vi "Mathcad 15 write file.vi"(8 "error in":errorcluster, 11 "DesignRequest":T1={"Project Folder"=path "", "Method Name"="", "Inputs"=[{"Label.Text"="L.Box", "Control Type"=0, "Numeric"=5.0, "Array"=[], "status"=FALSE, "Str Array"=[], "String"="", "unit"="m"}, {"Label.Text"="W.Box", "Control Type"=0, "Numeric"=2.0, "Array"=[], "status"=FALSE, "Str Array"=[], "String"="", "unit"="m"}, {"Label.Text"="H.Box", "Control Type"=0, "Numeric"=11.0, "Array"=[], "status"=FALSE, "Str Array"=[], "String"="", "unit"="m"}], "Version"=0}) -> (0 "error out":errorcluster, 3 "Mathcad w inputs":path)   [LabVIEW 2012, in "Design Server.lvlib"]
uses:
  Design Server.lvlib
  Design Request.ctl
  Variable cluster.ctl
  Folders.ctl
panel:
  out "file text":string
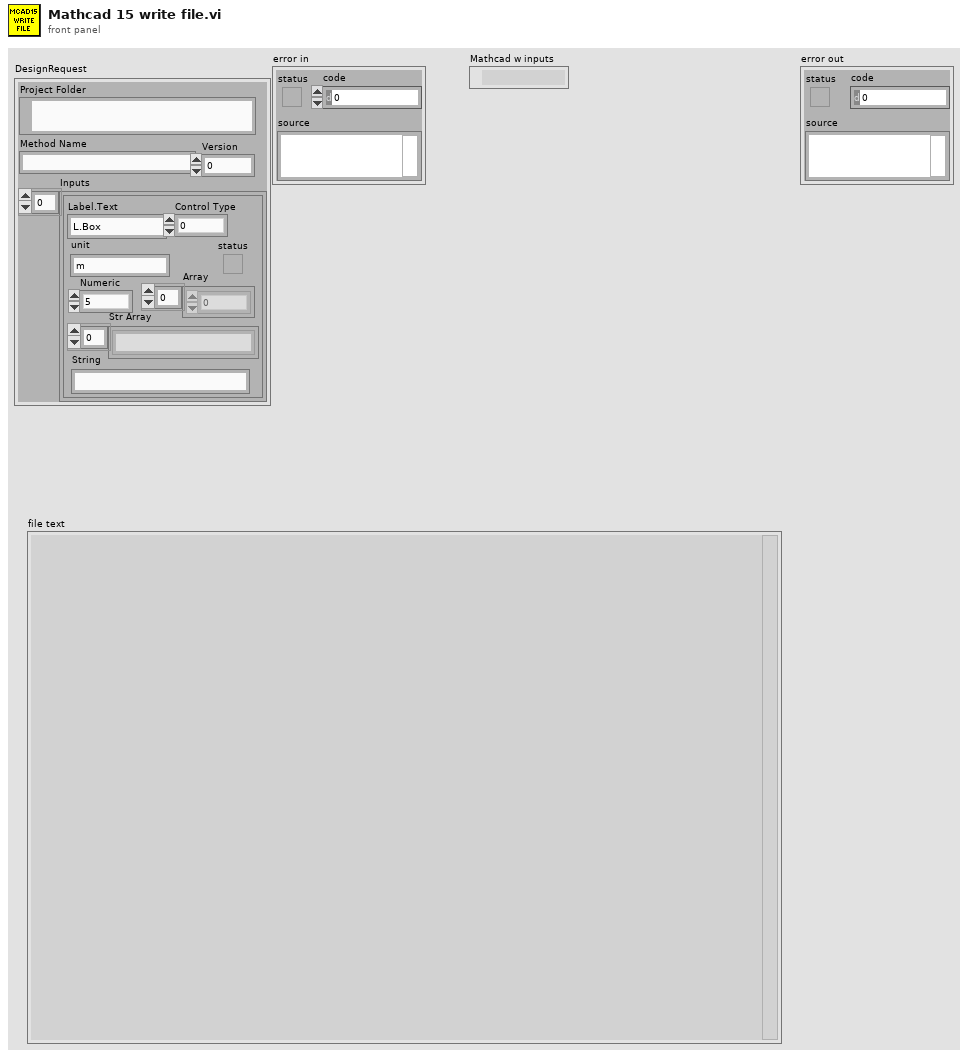
[diagram p1: front panel]
types:
  T1 = typedef "Design Server.lvlib/Design Request.ctl" = cluster{"Project Folder":path, "Method Name":string, "Inputs":T2, "Version":i32}
  T2 = typedef "Design Server.lvlib/Variable cluster.ctl" = cluster{"Label.Text":string, "Control Type":u32, "Numeric":dbl, "Array":dbl[], "status":bool, "Str Array":string[], "String":string, "unit":string}[]
  T3 = enum16{"open", "replace", "create", "open or create", "replace or create", "replace or create with confirmation"}
  T4 = typedef "Design Server.lvlib/Folders.ctl" = enum16{"MathcadMethods", "RequestedDesigns", "CompletedDesigns", "MathcadCode", "CollabnetSVN.exe"}
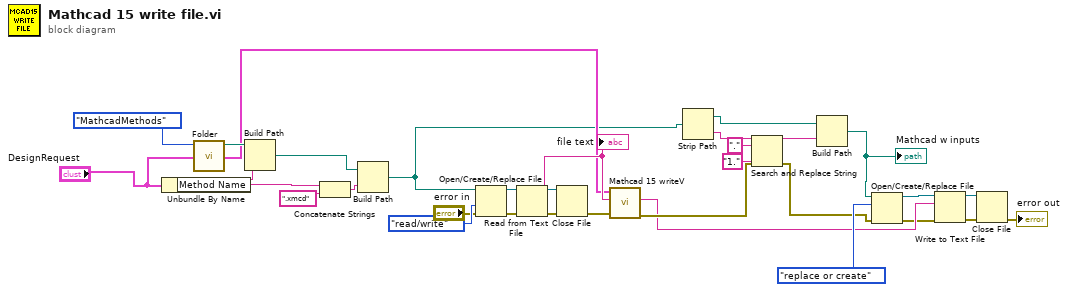
[diagram p0: block diagram]
diagram:
  n1 = Unbundle By Name("DesignRequest") -> ("Method Name"=w27:string)
  n2 = call "Folder.vi"("Folders"=Folders."MathcadMethods") -> ("FolderPath"=w28:path)  [unwired: 8 in, 2 out]
  n3 = Build Path(base path=w28, name or relative path=w27) -> (appended path=w23:path)
  n4 = Concatenate Strings(w27, ".xmcd" ("string")) -> (w30:string)
  n5 = Build Path(base path=w23, name or relative path=w30) -> (appended path=w1:path)
  n6 = Open/Create/Replace File(file path (use dialog)=w1, error in="error in", access (0:read/write)=enum16{"read/write", "read-only", "write-only"}."read/write") -> (refnum out=w26:refnum<file>, error out=w25:errorcluster)  [unwired: 3 in, 1 out]
  n7 = Read from Text File(file (use dialog)=w26, error in=w25) -> (refnum out=w18:refnum<file>, text=w22:string, error out=w20:errorcluster)  [unwired: 2 in, 1 out]
  "file text" <- w22
  n8 = Close File(refnum=w18, error in=w20) -> (error out=w19:errorcluster)  [unwired: 1 out]
  n9 = call "Mathcad 15 writeV.vi"("error in (no error)"=w19, "file text"=w22, "DesignRequest"="DesignRequest") -> ("error out"=w12:errorcluster, "file text out"=w7:string)  [unwired: 7 in]
  n10 = Strip Path(path=w1) -> (stripped path=w13:path, name=w17:string)
  n11 = Search and Replace String(input string=w17, search string=".", replace string="1." ("replace string (\"\")"), error in=w12) -> (result string=w14:string, error out=w9:errorcluster)  [unwired: 4 in, 2 out]
  n12 = Build Path(base path=w13, name or relative path=w14) -> (appended path=w11:path)
  "Mathcad w inputs" <- w11
  n13 = Open/Create/Replace File(file path (use dialog)=w11, error in=w9, operation (0:open)=T3."replace or create") -> (refnum out=w8:refnum<file>, error out=w6:errorcluster)  [unwired: 3 in, 1 out]
  n14 = Write to Text File(file (use dialog)=w8, text=w7, error in=w6) -> (refnum out=w4:refnum<file>, error out=w5:errorcluster)  [unwired: 1 in, 1 out]
  n15 = Close File(refnum=w4, error in=w5) -> (error out=→"error out":errorcluster)  [unwired: 1 out]
